vi "Devices.vi"() -> (3 "LINX Devices":string[][](array[string])=[["chipKIT Uno32", "chipKIT uC32", "chipKIT MAX32", "chipKIT dp32"]])   [LabVIEW 2011, in "LVH-LINX.lvlib" / "Device.lvlib"]
uses:
  Device.lvlib
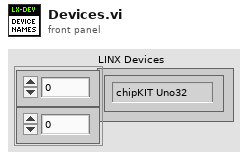
[diagram p1: front panel]
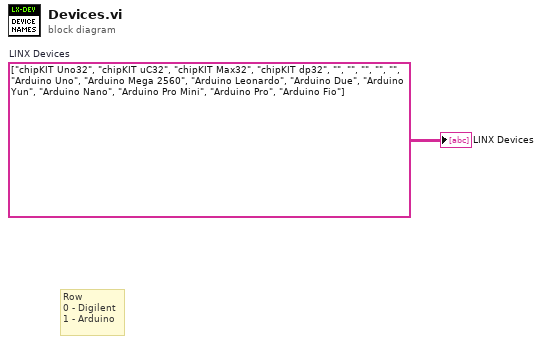
[diagram p0: block diagram]
diagram:
  w1 = string[][] [["chipKIT Uno32", "chipKIT uC32", "chipKIT Max32", "chipKIT dp32", "", "", "", "", ""], ["Arduino Uno", "Arduino Mega 2560", "Arduino Leonardo", "Arduino Due", "Arduino Yun", "Arduino Nano", "Arduino Pro Mini", "Arduino Pro", "Arduino Fio"]]  # LINX Devices
  # "Row\n0 - Digilent\n1 - Arduino"
  "LINX Devices" <- w1
